vi "split_XYZ_1D.vi"(0 "Point":dbl[](array[numeric])) -> (1 "X":dbl, 2 "Y":dbl, 3 "Z":dbl)   [LabVIEW 2015]
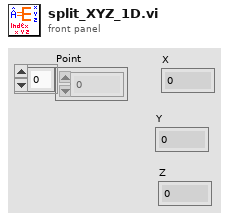
[diagram p1: front panel]
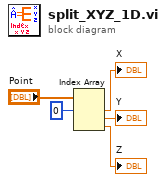
[diagram p0: block diagram]
diagram:
  n1 = Index Array(array="Point", index #1=0 ("index")) -> (element #1=→"X":dbl, element #2=→"Y":dbl, element #3=→"Z":dbl)  [unwired: 2 in]
